vi "SetLineStyle.vi"(0 "reference":refnum<class "SegmentedLineEdge.lvclass">, 1 "lineStyle":refnum<class "LineStyle.lvclass">, 5 "error in (no error)":errorcluster) -> (14 "reference out":refnum<class "SegmentedLineEdge.lvclass">, 19 "error out":errorcluster)   [LabVIEW 2012, in "SegmentedLineEdge.lvclass"]
doc: "Sets the line style property.\n @param newValue the new value\n\n public void setLineStyle(LineStyle newValue)"
uses:
  <resource>/Framework/Providers/Open_GDS/UML/SegmentedLineEdge_class/SegmentedLineEdge.lvclass
  <resource>/Framework/Providers/Open_GDS/UML/LineStyle_class/LineStyle.lvclass
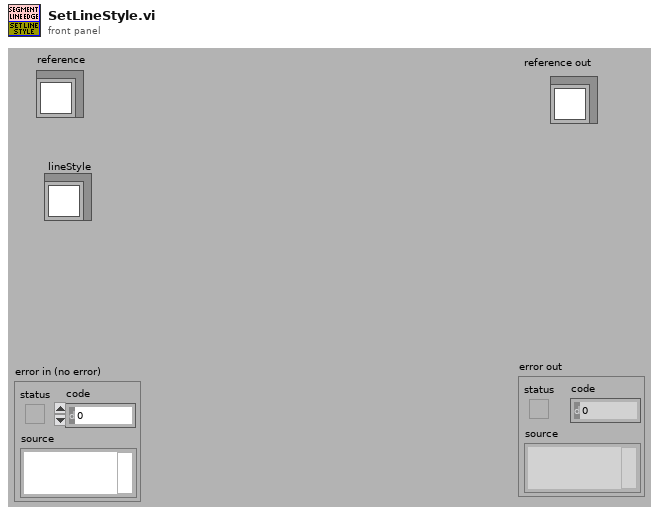
[diagram p1: front panel]
types:
  T1 = typedef "SegmentedLineEdge.lvclass/ObjectAttributes.ctl" = cluster{"Base class":T2, "lineStyle":refnum<class "LineStyle.lvclass">, "startArrowHead":refnum<class "ArrowHead.lvclass">, "endArrowHead":refnum<class "ArrowHead.lvclass">, "startLabel":string, "midLabel":string, "endLabel":string, "MidLabelOffset":T4, "SplitWire":bool}
  T2 = typedef "GeneralPathEdge.lvclass/ObjectAttributes.ctl" = cluster{"Base class":T3}
  T3 = typedef "AbstractEdge.lvclass/ObjectAttributes.ctl" = cluster{"start":refnum<class "AbstractNode.lvclass">, "end":refnum<class "AbstractNode.lvclass">}
  T4 = typedef "Point Point2D.ctl" = cluster{"x":dbl, "y":dbl}
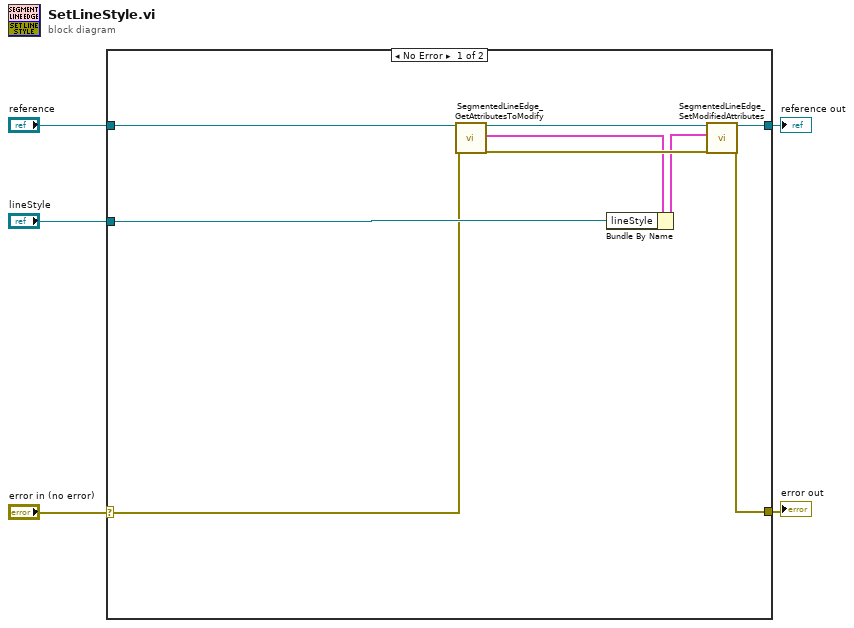
[diagram p0: block diagram]
diagram:
  n1 = case shown="No Error" "error in (no error)" {
    selector: "error in (no error)" -> [w6 w15]
    tunnel: "reference" -> [w14 w16]
    tunnel: [w13 w15] -> w4
    tunnel: [w12 w16] -> w3
    tunnel: "lineStyle" -> [w11 _]
    frame No Error {
      n2 = call <resource>:"SegmentedLineEdge_GetAttributesToModify.vi"("reference in"=w14, "error in (no error)"=w6) -> ("reference out"=w10:refnum<class "SegmentedLineEdge.lvclass">, "Attributes"=w8:T1, "error out"=w9:errorcluster)  [unwired: 1 in, 14 out]
      n3 = Bundle By Name(cluster=w8, "lineStyle"=w11) -> (w7:T1)
      n4 = call <resource>:"SegmentedLineEdge_SetModifiedAttributes.vi"("reference in"=w10, "Attributes"=w7, "error in (no error)"=w9) -> ("reference out"=w12:refnum<class "SegmentedLineEdge.lvclass">, "error out"=w13:errorcluster)  [unwired: 3 in, 12 out]
    }
    frame Error {
    }
  }
  "reference out" <- w3
  "error out" <- w4
